vi "SelectModel.vi"(0 "产品型号":string[](array[string])) -> (2 "当前零件型号":string, 3 "产品型号数据OK":bool)   [LabVIEW 2014]
panel:
  in  "Info":cluster{"机种型号":string, "确定":bool}
  # "请选择机种型号！"
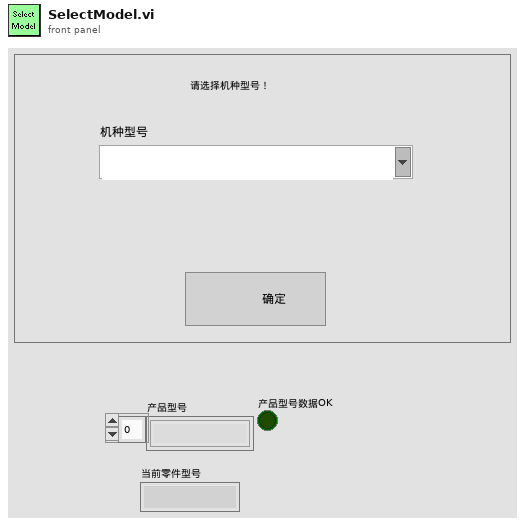
[diagram p1: front panel]
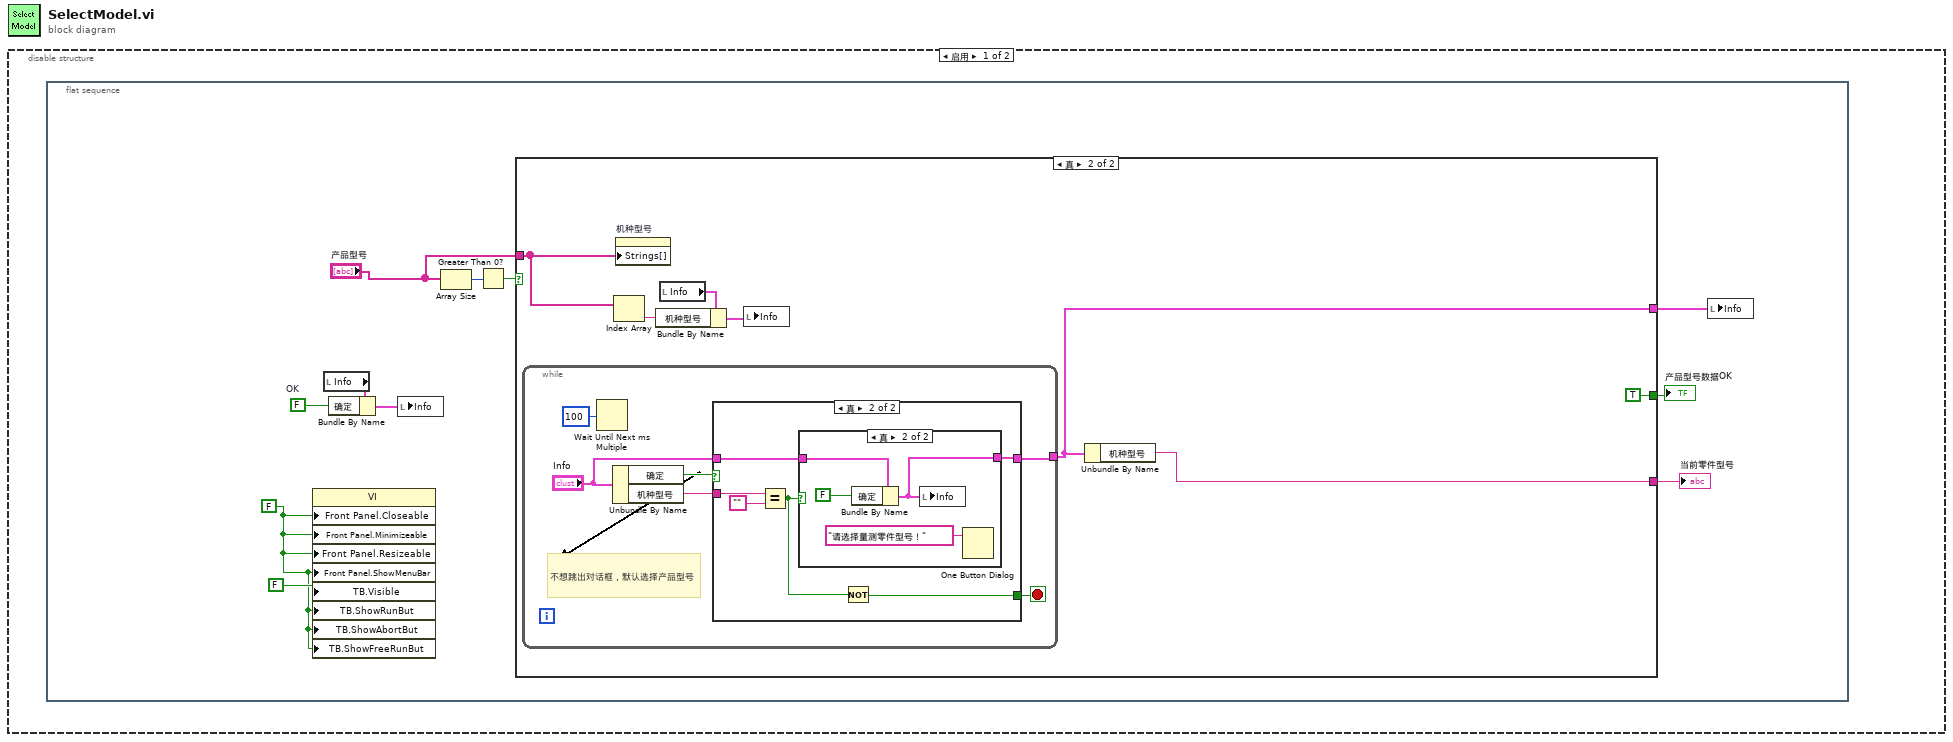
[diagram p0: block diagram]
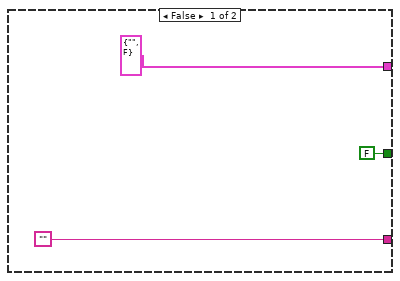
[diagram p2: hidden frame]
diagram:
  n1 = disable-structure shown="启用" {
    frame Enabled {
      n2 = flat-sequence {
        frame #0 {
          w6 = FALSE  # OK
          w1 = FALSE ("Front Panel Window:Closeable")
          n3 = property class="VI"("Front Panel.Closeable"=w1, "Front Panel.Minimizeable"=w1, "Front Panel.Resizeable"=w1, "Front Panel.ShowMenuBar"=w1, "TB.Visible"=FALSE ("工具栏:可见"), "TB.ShowRunBut"=w1, "TB.ShowAbortBut"=w1, "TB.ShowFreeRunBut"=w1) -> ()  [unwired: 2 in, 2 out]
          n4 = local read "Info"() -> (w5:cluster{"机种型号":string, "确定":bool})
          n5 = Bundle By Name(cluster=w5, "确定"=w6) -> (w7:cluster{"机种型号":string, "确定":bool})
          n6 = local write "Info"(w7) -> ()
          n7 = Array Size(array="产品型号") -> (size(s)=w10:i32)
          n8 = Greater Than 0?(x=w10) -> (x > 0?=w9:bool)
          n9 = case shown="真" w9 {
            tunnel: [cluster{"机种型号":string, "确定":bool} {"机种型号"="", "确定"=FALSE} ("Info") w20] -> w11
            tunnel: ["" w19] -> w8
            tunnel: [FALSE TRUE] -> w4
            tunnel: "产品型号" -> [_ w16]
            frame False {
            }
            frame True {
              n10 = while {
                tunnel: [w25] -> w20
                stop <- w26 stop-if-true
                # "不想跳出对话框，默认选择产品型号"
                n11 = Wait Until Next ms Multiple(millisecond multiple=i64 100 ("Period")) -> ()  [unwired: 1 out]
                n12 = Unbundle By Name("Info") -> ("确定"=w22:bool, "机种型号"=w23:string)
                n13 = case shown="真" w22 {
                  selector: w22 -> [w29 _]
                  tunnel: [w29 w35] -> w26
                  tunnel: "Info" -> [w28 w32]
                  tunnel: [w28 w31] -> w25
                  tunnel: w23 -> [_ w30]
                  frame False {
                  }
                  frame True {
                    n14 = Equal?(x=w30, y="") -> (x = y?=w33:bool)
                    n15 = case shown="真" w33 {
                      tunnel: w32 -> [w36 w39]
                      tunnel: [w36 w37] -> w31
                      frame False {
                      }
                      frame True {
                        n16 = Bundle By Name(cluster=w39, "确定"=FALSE ("确定按钮")) -> (w37:cluster{"机种型号":string, "确定":bool})
                        n17 = local write "Info"(w37) -> ()
                        n18 = One Button Dialog(message="请选择量测零件型号！" ("消息")) -> ()  [unwired: 1 in, 1 out]
                      }
                    }
                    n19 = Not(x=w33) -> (.not. x?=w35:bool)
                  }
                }
              }
              n20 = Index Array(array=w16) -> (element=w15:string)  [unwired: 1 in]
              n21 = property on="机种型号" class="CmbBox"("Strings[]"=w16) -> ()  [unwired: 2 in, 2 out]
              n22 = local read "Info"() -> (w21:cluster{"机种型号":string, "确定":bool})
              n23 = Bundle By Name(cluster=w21, "机种型号"=w15) -> (w18:cluster{"机种型号":string, "确定":bool})
              n24 = local write "Info"(w18) -> ()
              n25 = Unbundle By Name(w20) -> ("机种型号"=w19:string)
            }
          }
          "当前零件型号" <- w8
          "产品型号数据OK" <- w4
          n26 = local write "Info"(w11) -> ()
        }
      }
    }
    frame Disabled {
    }
  }
